vi "X_rails_DF2.vi"() -> ()   [LabVIEW 2019]
panel:
  in  "STOP SM":bool
  in  "X":dbl=-5.75
  in  "nb of iteration":dbl=100.0
  in  "F1 normal speed":dbl=85.0
  in  "RUN PRINT":bool
  in  "Stop program":bool
  # "HOW TO STOP THE STEPPER MOTOR"
  # "Press 'STOP SM' then 'Stop program' to stop the labview program"
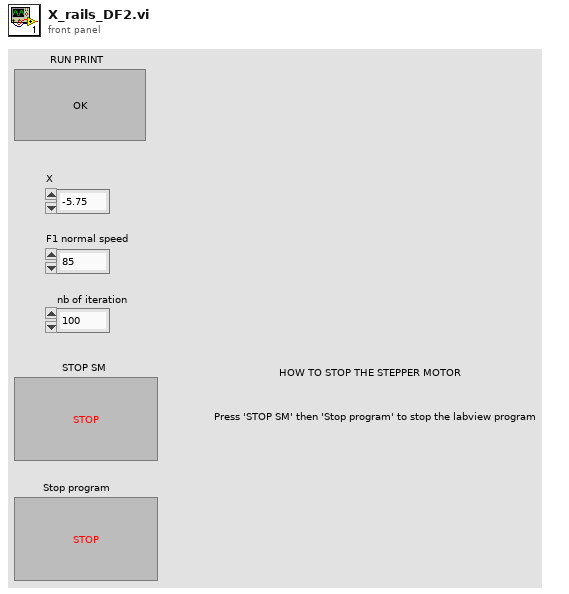
[diagram p1: front panel]
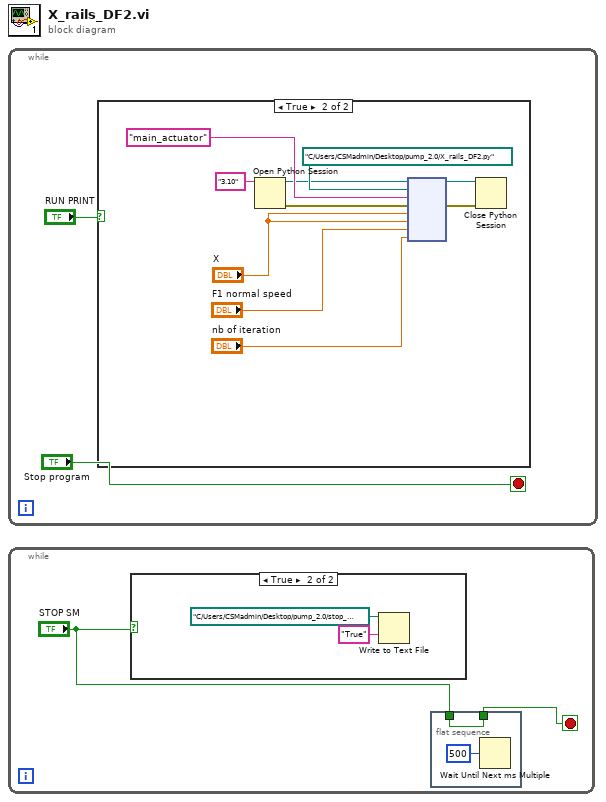
[diagram p0: block diagram]
diagram:
  n1 = while {
    stop <- "Stop program" stop-if-true
    n2 = case shown="True" "RUN PRINT" {
      frame False {
      }
      frame True {
        n3 = Open Python Session(python version="3.10" ("Python version")) -> (session out=w6:refnum<k35>, error out=w5:errorcluster)  [unwired: 2 in]
        n4 = node(w6, path "C:/Users/CSMadmin/Desktop/pump_2.0/X_rails_DF2.py" ("module path"), "main_actuator" ("function name"), w5, "X", "X", "F1 normal speed", "nb of iteration") -> (w11:refnum<k35>, w10:errorcluster)  [unwired: 4 in, 2 out]
        n5 = Close Python Session(session in=w11, error in=w10) -> ()  [unwired: 1 out]
      }
    }
  }
  n6 = while {
    stop <- w13 stop-if-true
    n7 = case shown="True" "STOP SM" {
      frame False {
      }
      frame True {
        n8 = Write to Text File(file (use dialog)=path "C:/Users/CSMadmin/Desktop/pump_2.0/stop_cache.txt", text="True") -> ()  [unwired: 2 in, 3 out]
      }
    }
    n9 = flat-sequence {
      tunnel: "STOP SM" -> [w15]
      tunnel: [w15] -> w13
      frame #0 {
        n10 = Wait Until Next ms Multiple(millisecond multiple=u32 500) -> ()  [unwired: 1 out]
      }
    }
  }
